vi "AssetInterface_Update Tags.vi"(8 "error in (no error)":errorcluster, 10 "TagBus DVR":refnum<data-value>, 11 "Asset_Interface in":refnum<class "EnergyStorage.lvclass">) -> (0 "error out":errorcluster, 2 "TagBus DVR out":refnum<data-value>, 3 "Asset_Interface out":refnum<class "EnergyStorage.lvclass">)   [LabVIEW 2015, in "EnergyStorage.lvclass"]
uses:
  EnergyStorage.lvclass
  TagBus/TagBus.lvclass
  EnergyStorage.lvclass/EnergyStorage.ctl
panel:
  out "Status":cluster{"kW":dbl}
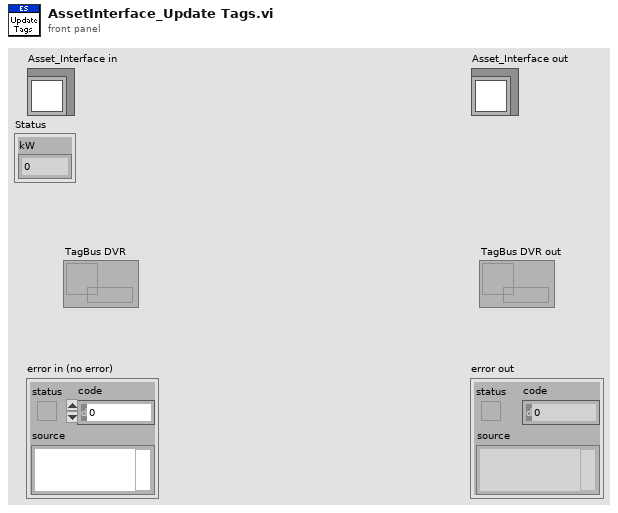
[diagram p1: front panel]
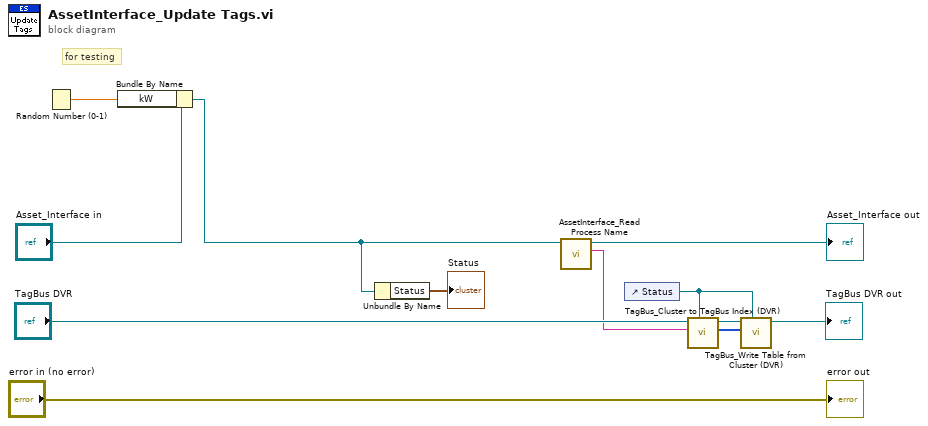
[diagram p0: block diagram]
diagram:
  # "for testing"
  n1 = Random Number (0-1)() -> (number: 0 to 1=w7:dbl)
  n2 = Bundle By Name(cluster="Asset_Interface in", "kW"=w7) -> (w8:refnum<class "EnergyStorage.lvclass">)
  n3 = Unbundle By Name(w8) -> ("Status"=→"Status":cluster{"kW":dbl})
  n4 = call-dynamic "AssetInterface_Read Process Name.vi"("EnergyStorage in"=w8) -> ("Process Name"=w1:string, "EnergyStorage out"=→"Asset_Interface out":refnum<class "EnergyStorage.lvclass">)  [unwired: 9 in]
  n5 = control-ref of="Status"() -> (w3:refnum<vi>)
  n6 = call "TagBus_Cluster to TagBus Index (DVR).vi"("Clust Refnum"=w3, "Tag Name Prepend"=w1, "TagBus DVR"="TagBus DVR") -> ("Index Array"=w4:i32[], "TagBus DVR out"=w5:refnum<data-value>)  [unwired: 7 in]
  n7 = call "TagBus_Write Table from Cluster (DVR).vi"("Clust Refnum"=w3, "Index Array"=w4, "Data Value Reference in"=w5) -> ("Data Value Reference out"=→"TagBus DVR out":refnum<data-value>)  [unwired: 8 in]
  "error out" <- "error in (no error)"
